vi "Launch.vi"(8 "error in (no error)":errorcluster, 11 "Zero Timeout Message Handler in":refnum<class "Zero Timeout Message Handler.lvclass">) -> (0 "error out":errorcluster, 3 "Message Queue":refnum<queue>)   [LabVIEW 2024, in "Zero Timeout Message Handler.lvlib" / "Zero Timeout Message Handler.lvclass"]
uses:
  Zero Timeout Message Handler.lvclass
  ~Message/~Message.lvclass
  Main.vi
  Zero Timeout Message Handler.lvclass/Zero Timeout Message Handler.ctl
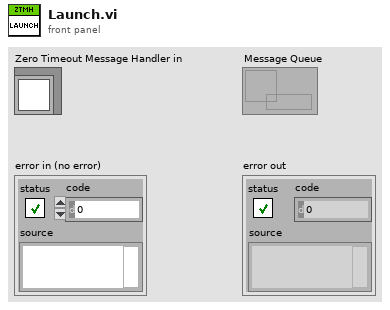
[diagram p1: front panel]
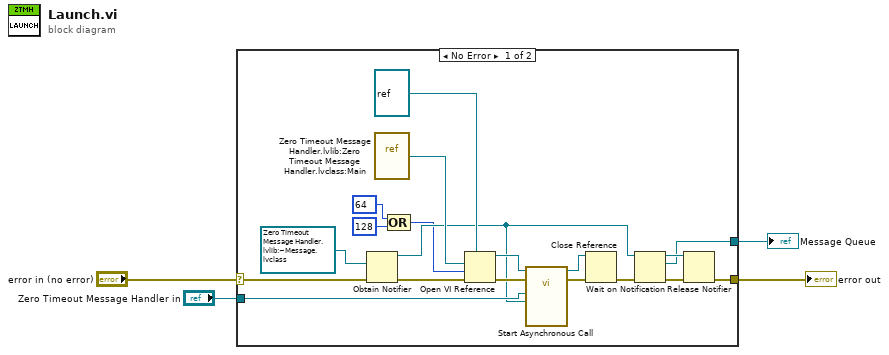
[diagram p0: block diagram]
diagram:
  n1 = case shown="No Error" "error in (no error)" {
    selector: "error in (no error)" -> [w14 w24]
    tunnel: [w8 w24] -> w3
    tunnel: "Zero Timeout Message Handler in" -> [w19 _]
    tunnel: [w6 _] -> w1
    frame No Error {
      n2 = Obtain Notifier(notification data type=refnum<queue> refnum ("queue out"), error in (no error)=w14) -> (notifier out=w11:refnum<notifier>, error out=w13:errorcluster)  [unwired: 2 in, 1 out]
      n3 = vi-ref "Zero Timeout Message Handler.lvlib:Zero Timeout Message Handler.lvclass:Main.vi"() -> (w23:refnum<vi>)
      n4 = Compound Arithmetic op=OR(64, 128) -> (w5:i32)
      n5 = Open VI Reference(type specifier VI Refnum (for type only)=refnum<vi> refnum, vi path=w23, options=w5, error in (no error)=w13) -> (vi reference=w20:refnum<vi>, error out=w18:errorcluster)  [unwired: 2 in]
      n6 = call-by-ref "Start Asynchronous Call"(reference=w20, error in=w18, "Message Queue Notifier"=w11, "Zero Timeout Message Handler in"=w19) -> (reference out=w16:refnum<vi>, error out=w17:errorcluster)  [unwired: 10 in]
      n7 = Close Reference(reference=w16, error in (no error)=w17) -> (error out=w12:errorcluster)
      n8 = Wait on Notification(notifier=w11, error in (no error)=w12) -> (notifier out=w7:refnum<notifier>, notification=w6:refnum<queue>, error out=w9:errorcluster)  [unwired: 2 in, 1 out]
      n9 = Release Notifier(notifier=w7, error in (no error)=w9) -> (error out=w8:errorcluster)  [unwired: 1 in, 2 out]
    }
    frame Error {
    }
  }
  "error out" <- w3
  "Message Queue" <- w1
